vi "TargetArduinoControlled.vi"() -> ()   [LabVIEW 2013]
uses:
  <vilib>/Instr/_visa.llb/VISA Configure Serial Port (Instr).vi
  <vilib>/express/express arith-compare/Formula/XNode/ExpressFormulaBlockNode.xnode
panel:
  out "Tension de commande (V)":dbl
  out "Phidget device handle 2":i64
  out "Phidget device handle":i64
  out "Phidget Error Cluster":errorcluster
  in  "ArduinoSpeedSelect":i8(slide) scale=0.0..3.0
  out "Arduino Answer":string
  in  "Test Function":bool
  in  "Calibrate":bool
  out "shot until":dbl
  out "Target":cluster{dbl, dbl}(knob)={0.0, 360.0} scale=0.0..360.0
  in  "Shoot":bool
  out "TargetPosition":dbl
  out "moving":bool
  in  "Continious Slow motion":bool
  in  "Reset Shots":bool
  in  "Stop":bool
  in  "VISA resource name":refnum<visa-resource-name>="COM7" caption="Arduino Communication Port"
  out "shooting length (mm)":dbl
  in  "Sequence (ms)":i16
  in  "start rotation":bool
  in  "rotation stop":bool
  out "shooting radius (microns)":dbl
  in  "target radius":dbl=50600.0
  in  "Spot_spacing_µm":dbl=100.0
  in  "Position edge (microns)":dbl=-8706.0
  in  "Position Target (microns)":dbl=14475.0
  out "SpeedTarget  (rounds/s)":dbl
  out "tension envoyée V":dbl
  in  "event trigger":bool
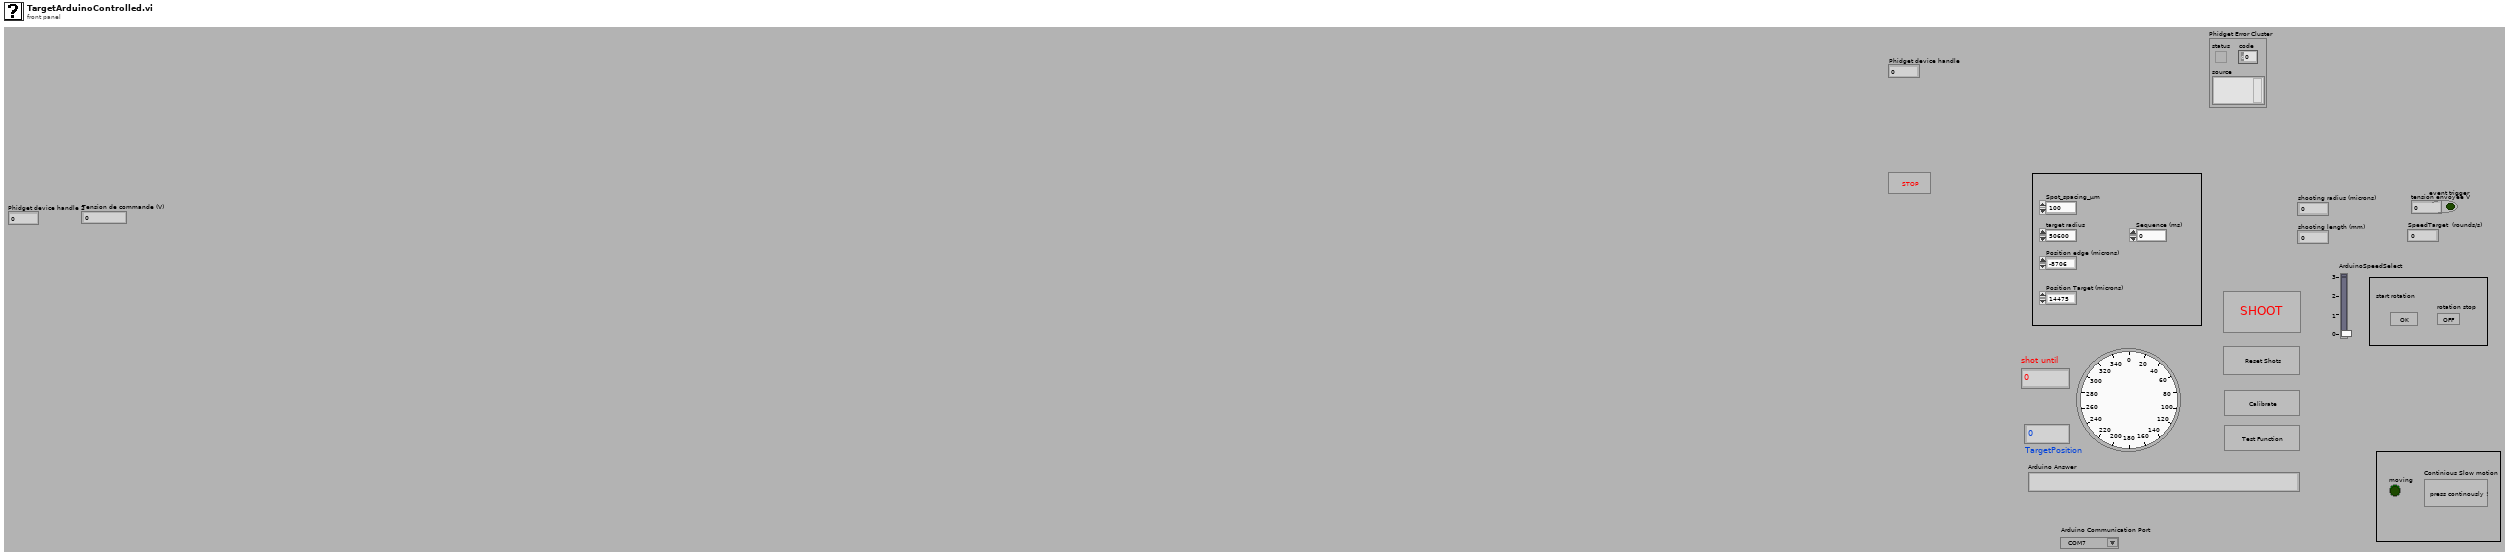
[diagram p1: front panel]
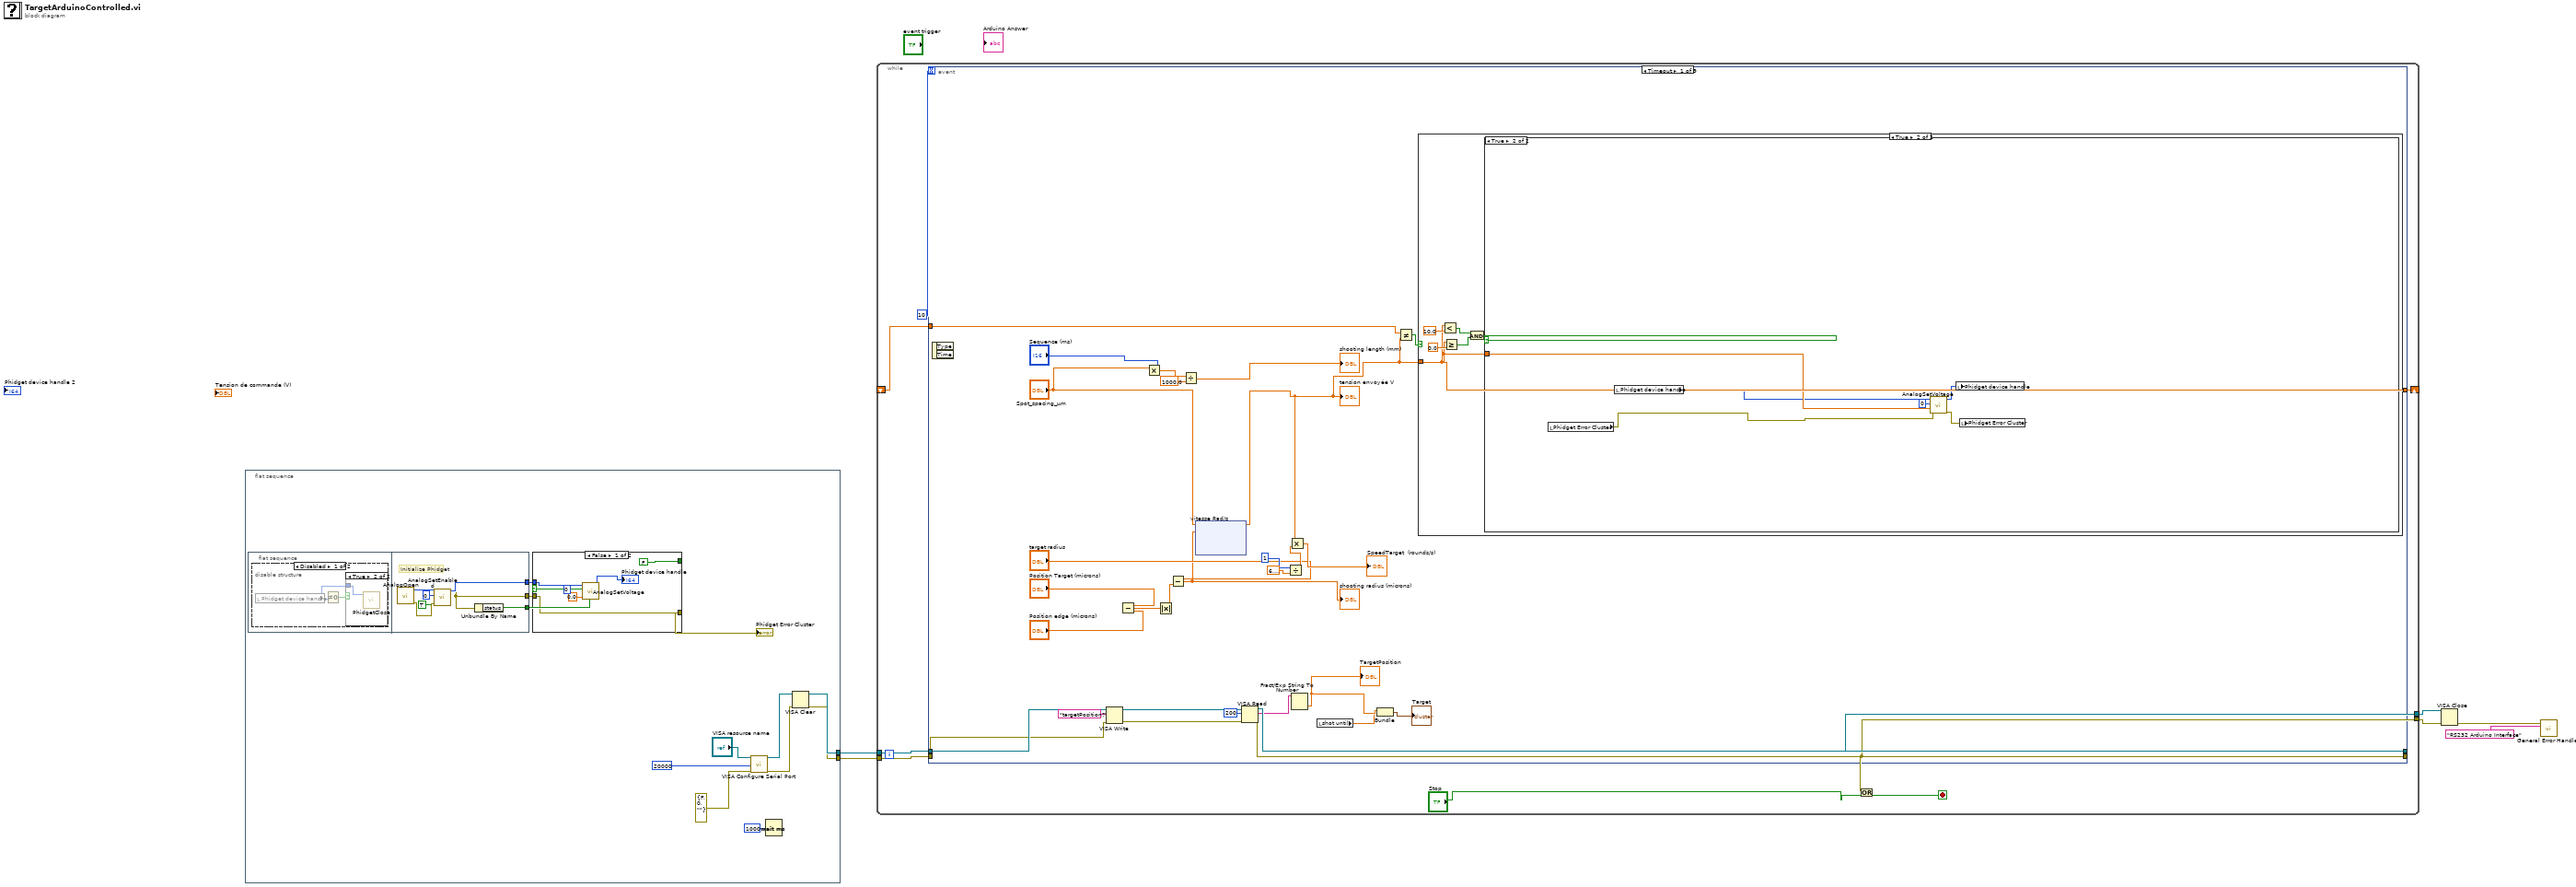
[diagram p0: block diagram]
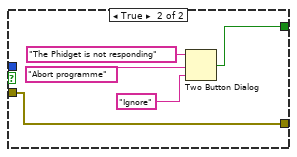
[diagram p2: hidden frame]
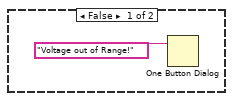
[diagram p6: hidden frame]
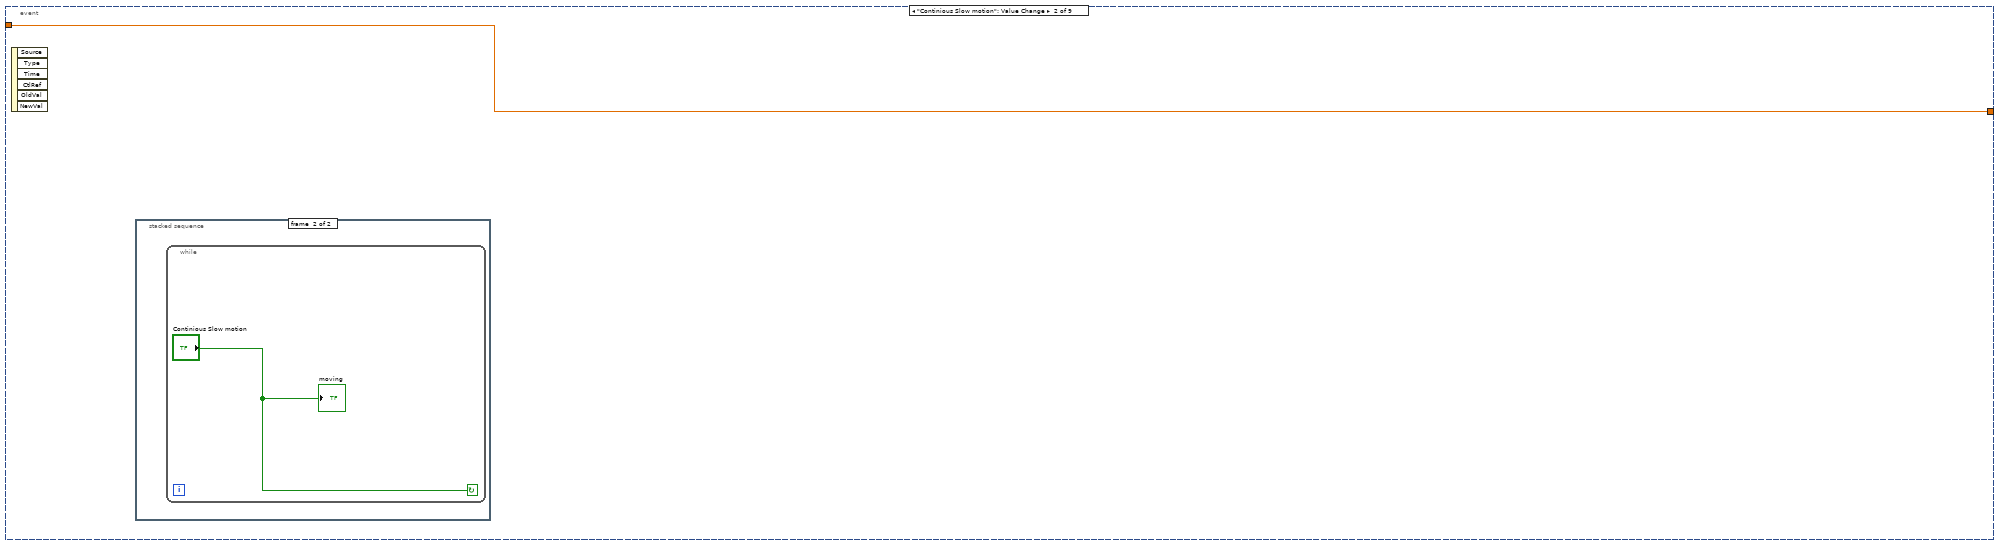
[diagram p7: hidden frame]
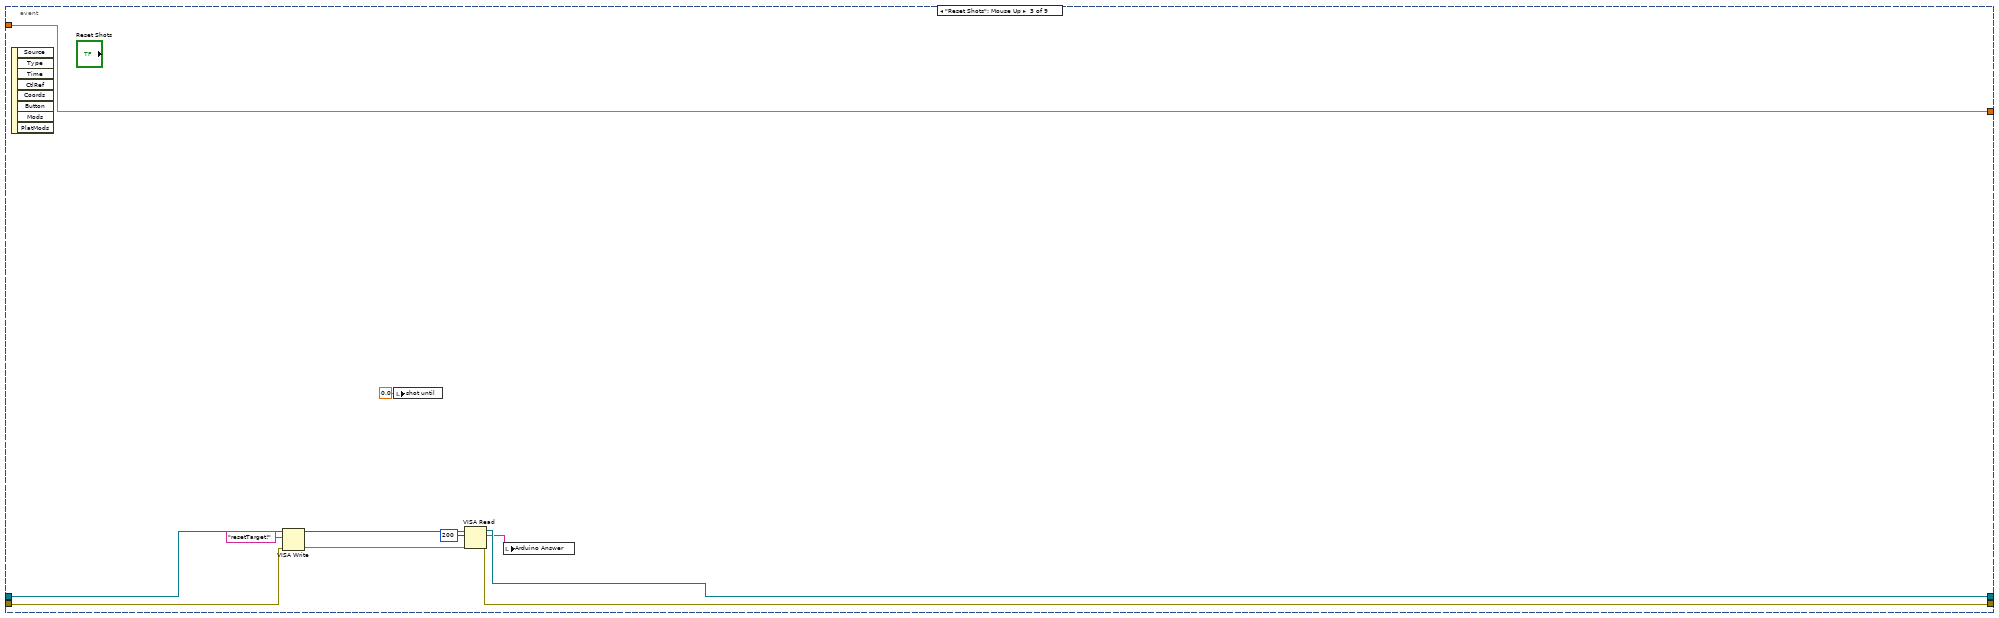
[diagram p9: hidden frame]
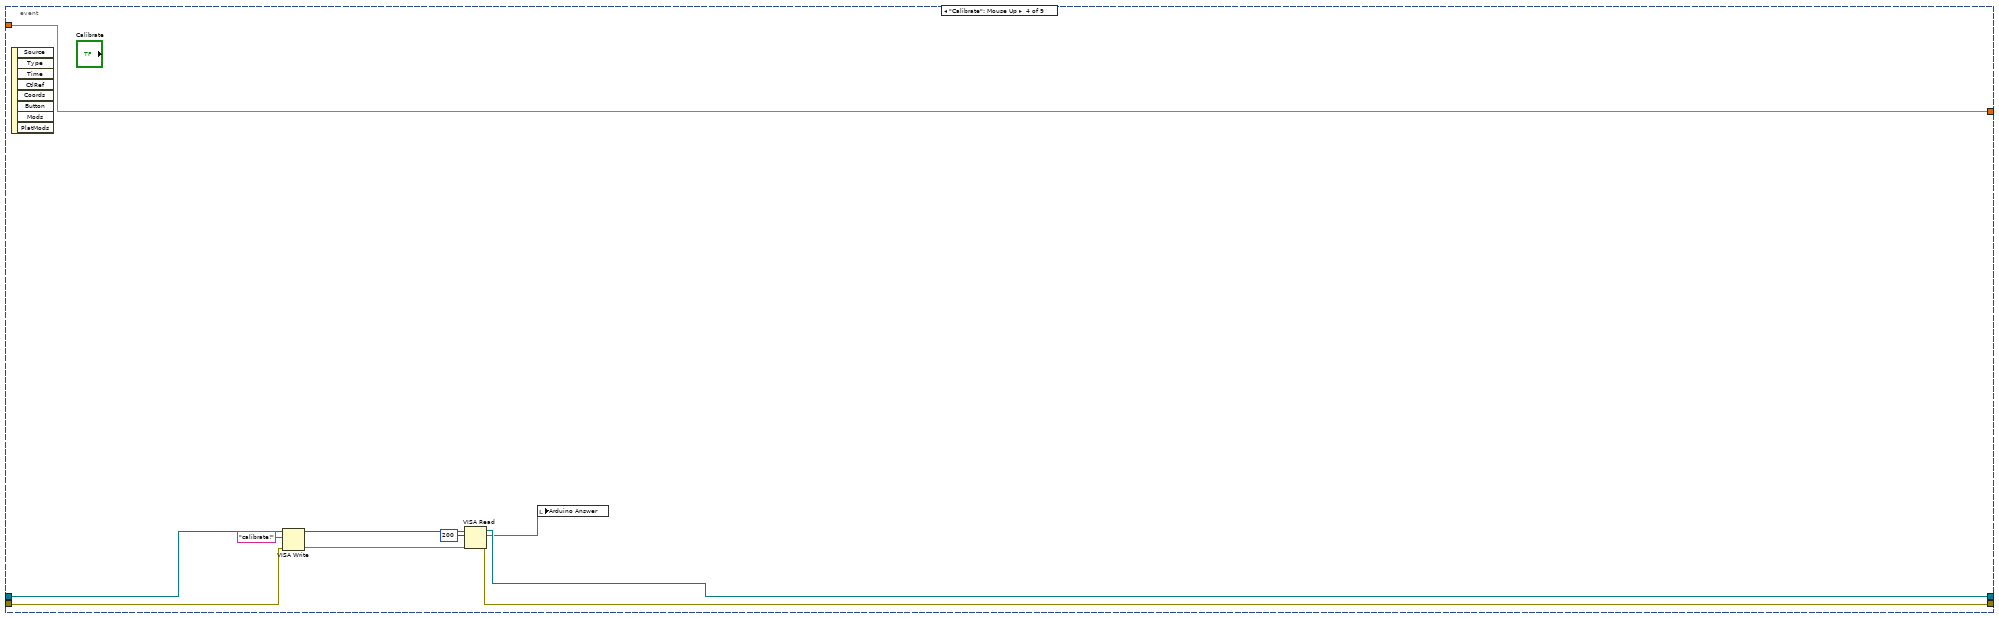
[diagram p10: hidden frame]
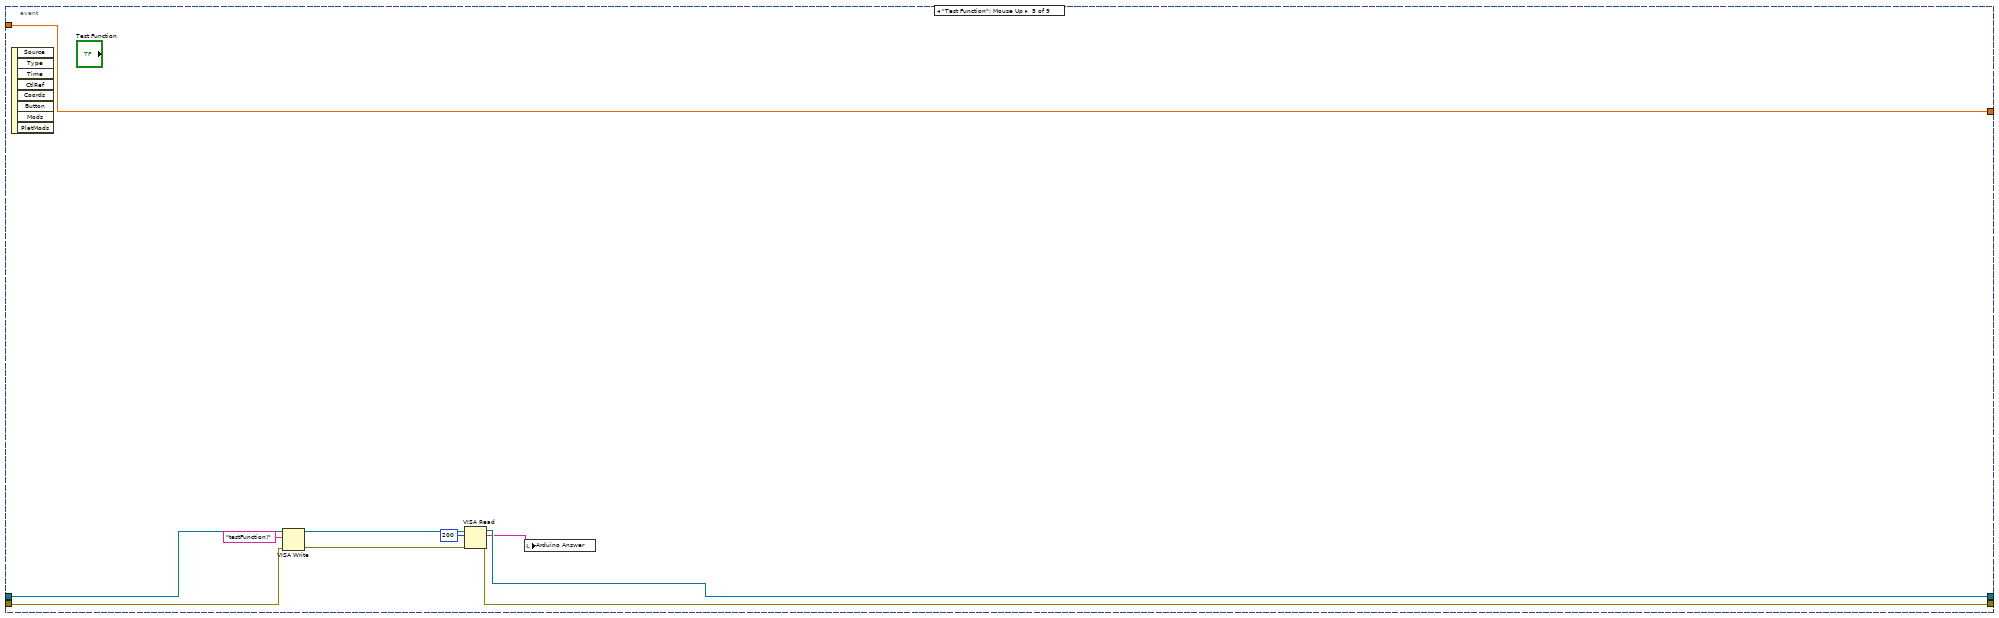
[diagram p11: hidden frame]
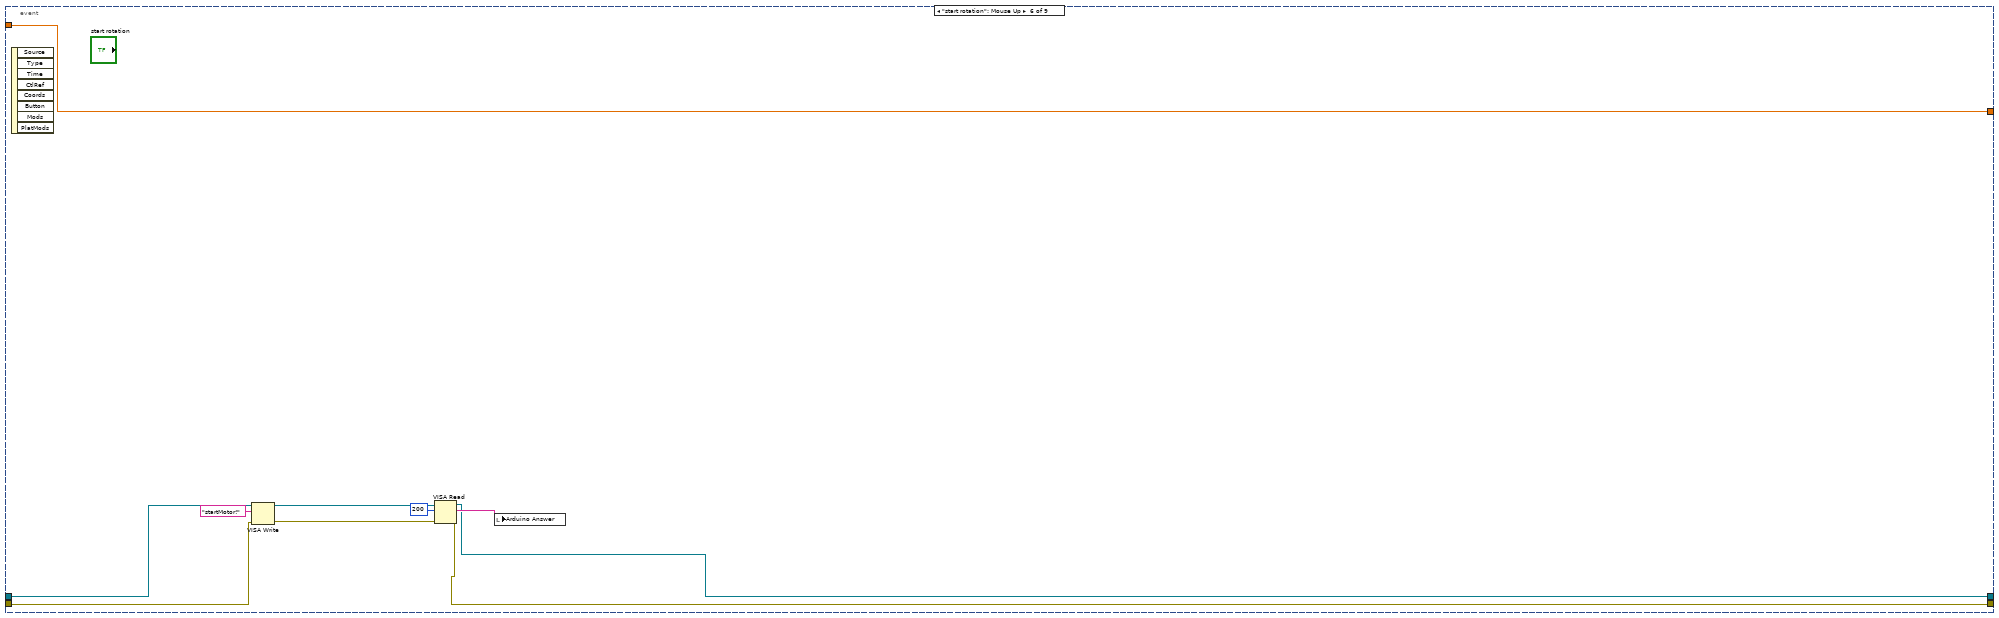
[diagram p12: hidden frame]
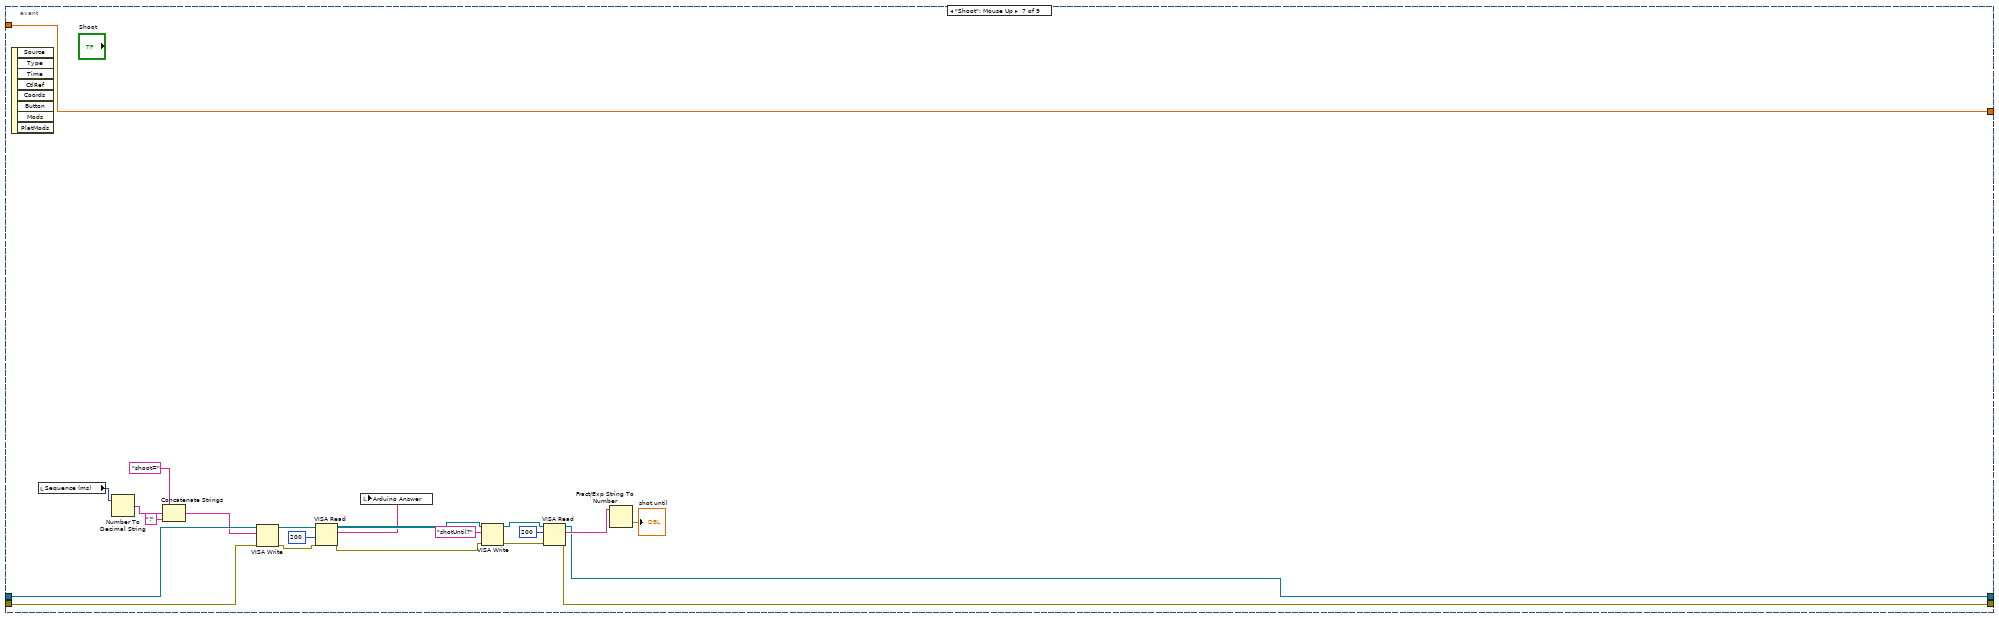
[diagram p13: hidden frame]
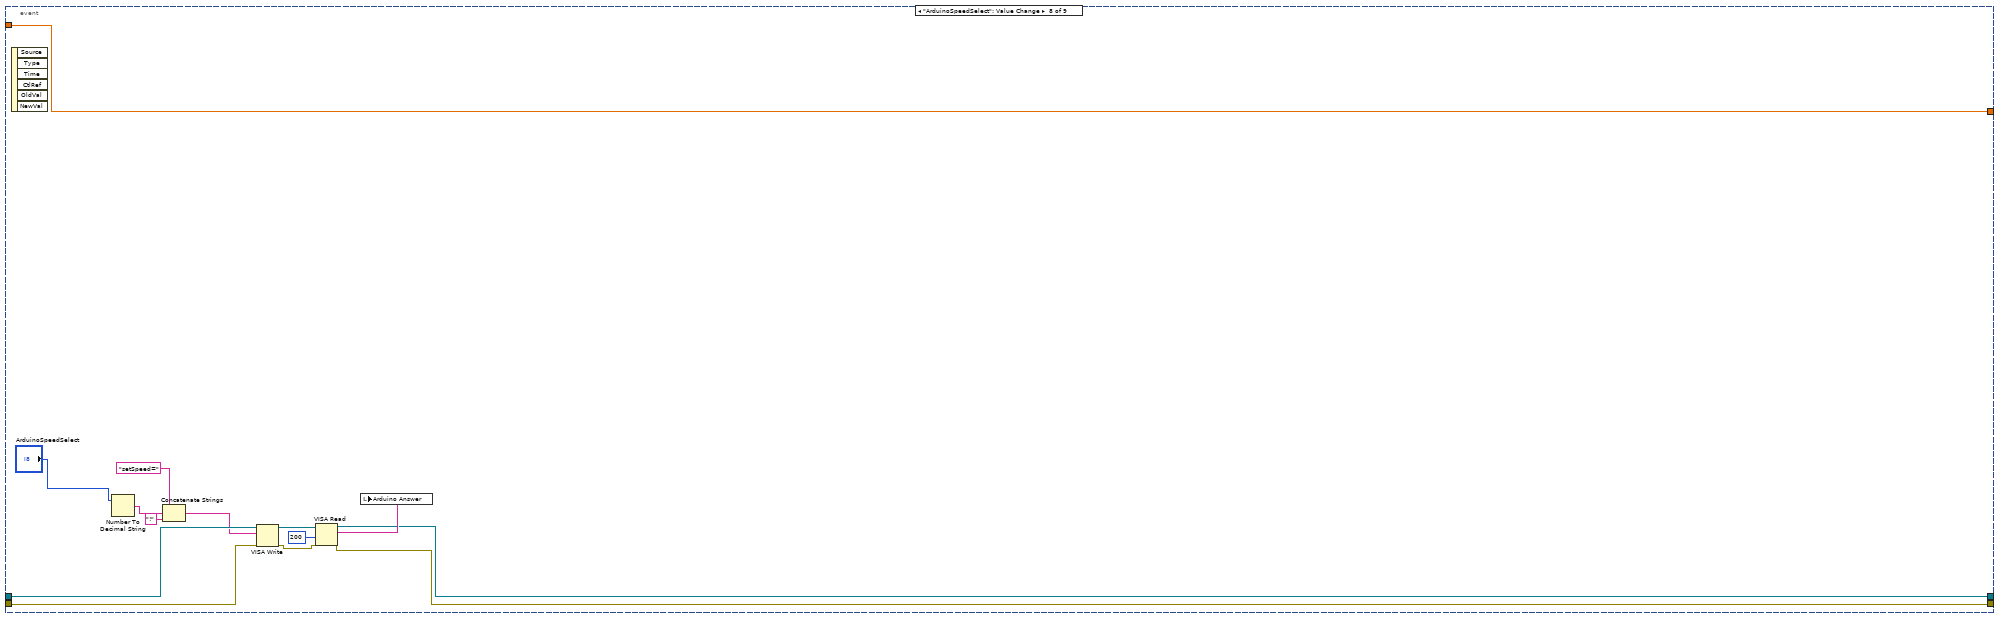
[diagram p14: hidden frame]
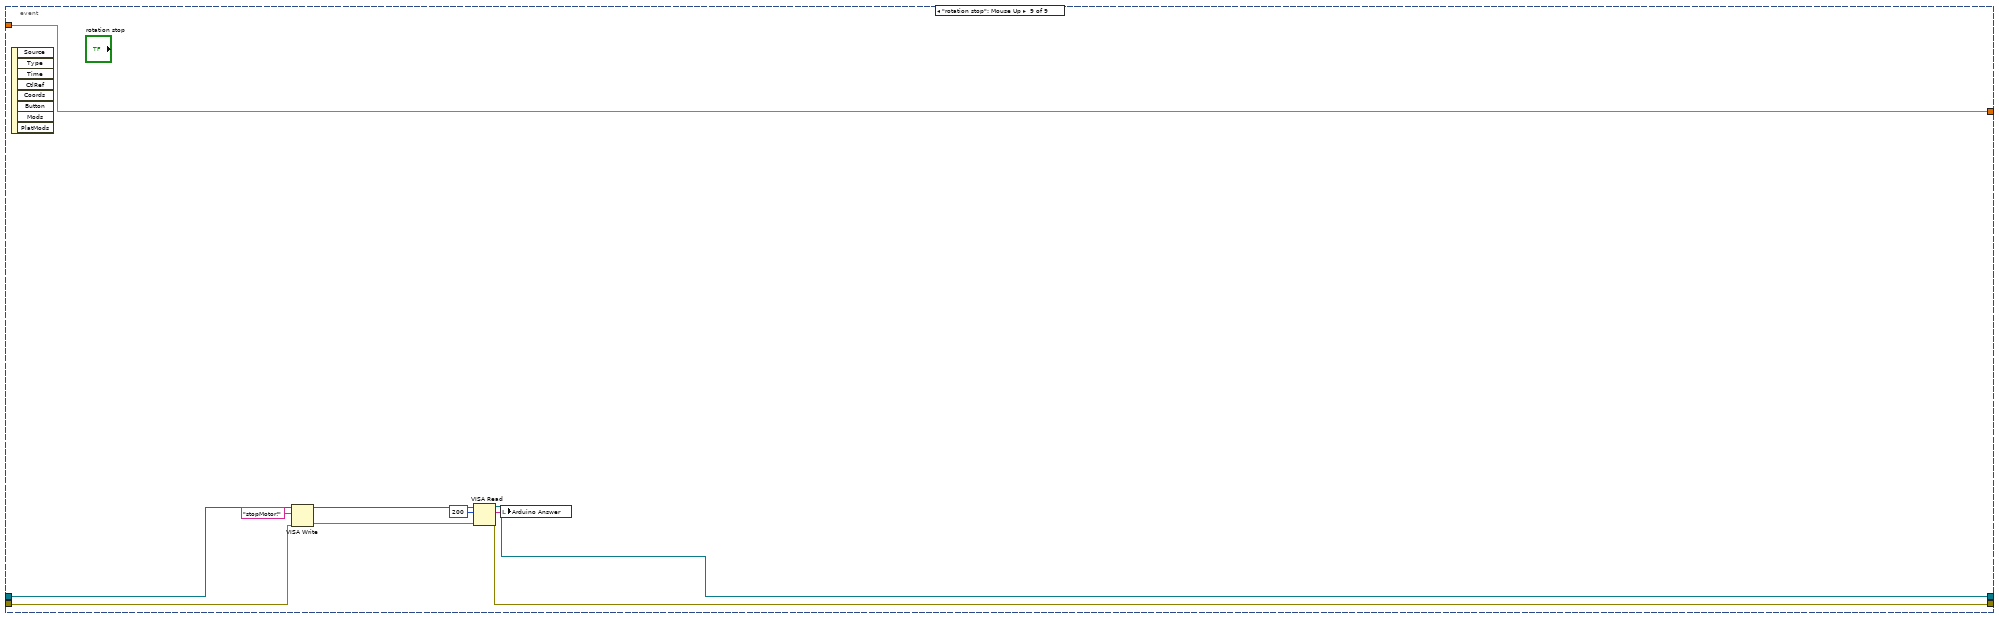
[diagram p15: hidden frame]
diagram:
  n1 = flat-sequence {
    tunnel: [w13] -> w6
    tunnel: [w12] -> w5
    frame #0 {
      n2 = flat-sequence {
        tunnel: [w35] -> w8
        tunnel: [w34] -> w9
        tunnel: [w33] -> w10
        frame #0 {
          n3 = disable-structure shown="Disabled" {
            frame Disabled {
              n4 = local read "Phidget device handle"() -> (w30:i64)
              n5 = Not Equal To 0?(x=w30) -> (x != 0?=w31:bool)
              n6 = case shown="True" w31 {
                tunnel: w30 -> [_ w32]
                frame False {
                }
                frame True {
                  n7 = call "PhidgetClose.vi"("Device In"=w32) -> ()  [unwired: 10 in, 1 out]
                }
              }
            }
            frame Enabled {
            }
          }
        }
        frame #1 {
          # "Initialize Phidget"
          n8 = call "AnalogOpen.vi"() -> ("error out"=w39:errorcluster, "Device Out"=w36:i32)  [unwired: 8 in, 2 out]
          n9 = call "AnalogSetEnabled.vi"("error in (no error)"=w39, "SetEnabled"=TRUE, "index"=0, "Device In"=w36) -> ("error out"=w33:errorcluster, "Device Out"=w34:i32)  [unwired: 5 in]
          n10 = Unbundle By Name(w33) -> ("status"=w35:bool)
        }
      }
      n11 = case shown="False" w8 {
        tunnel: [FALSE w26] -> _
        tunnel: w9 -> [w23 _]
        tunnel: w10 -> [w21 w25]
        tunnel: [w21 w25] -> w7
        frame False {
          n12 = call "AnalogSetVoltage.vi"("voltage"=0.0, "index"=0, "Device In"=w23) -> ("Device Out"=→"Phidget device handle":i32)  [unwired: 6 in, 1 out]
        }
        frame True {
          n13 = Two Button Dialog(message="The Phidget is not responding", 1:"Ignore" ("Nom du bouton V (\"OK\")"), 2:"Abort programme" ("Nom du bouton V (\"OK\")")) -> (T button?=w26:bool)
        }
      }
      "Phidget Error Cluster" <- w7
      n14 = call-poly "VISA Configure Serial Port"("VISA resource name"="VISA resource name", "timeout (10sec)"=u32 20000, "error in (no error)"=errorcluster {"status"=FALSE, "code"=0, "source"=""}) -> ("VISA resource name out"=w16:refnum<visa-resource-name>, "error out"=w14:errorcluster)  [unwired: 11 in]
      n15 = Wait (ms)(milliseconds to wait=u32 1000 ("attente (ms)")) -> ()  [unwired: 1 out]
      n16 = VISA Clear(VISA resource name=w16, error in (no error)=w14) -> (VISA resource name out=w13:refnum<visa-resource-name>, error out=w12:errorcluster)
    }
  }
  n17 = while {
    tunnel: w6 -> [w46]
    tunnel: w5 -> [w45]
    tunnel: [w42] -> w3
    tunnel: [w44] -> w2
    shift-right: [w41] -> _
    shift-left: _ -> [w40]
    stop <- w43 stop-if-true
    n18 = event shown="[0] Timeout" {
      selector: _ -> [_ _ _ _ _ _ _ _ _]
      dyn-events: _ -> [_ _ _ _ _ _ _ _ _]
      timeout: 10 -> [_ _ _ _ _ _ _ _ _]
      tunnel: w46 -> [w64 _ w110 w120 w130 w139 w162 w180 w183]
      tunnel: [w62 _ w108 w118 w128 w137 w164 w170 w185] -> w44
      tunnel: [w61 _ w107 w117 w127 w136 w163 w169 w184] -> w42
      tunnel: w45 -> [w59 _ w109 w119 w129 w138 w161 w179 w182]
      tunnel: [w50 w102 w104 w115 w125 w135 w145 w167 w181] -> w41
      tunnel: w40 -> [w51 w102 w104 w115 w125 w135 w145 w167 w181]
      event Timeout {
        n19 = event-data() -> ()  [unwired: 1 in, 2 out]
        n20 = VISA Write(VISA resource name=w64, write buffer="targetPosition?" ("buffer à écrire"), error in (no error)=w59) -> (VISA resource name out=w63:refnum<visa-resource-name>, error out=w60:errorcluster)  [unwired: 1 out]
        n21 = Subtract(x="Position Target (microns)", y="Position edge (microns)") -> (x-y=w73:dbl)
        n22 = Multiply(x="Spot_spacing_µm", y="Sequence (ms)") -> (x*y=w68:dbl)
        n23 = Absolute Value(x=w73) -> (abs(x)=w72:dbl)
        n24 = Subtract(x="target radius", y=w72) -> (x-y=w65:dbl)
        "shooting radius (microns)" <- w65
        n25 = Divide(x=w68, y=1000.0) -> (x/y=→"shooting length (mm)":dbl)
        n26 = xnode ("vitesse Rad/s")("Spot_spacing_µm"="Spot_spacing_µm", "Radius_µm"=w65) -> ("Result"=w50:dbl)  [unwired: 1 in, 1 out]
        "tension envoyée V" <- w50
        n27 = VISA Read(VISA resource name=w63, byte count=u32 200 ("nombre d'octets"), error in (no error)=w60) -> (VISA resource name out=w62:refnum<visa-resource-name>, read buffer=w56:string, error out=w61:errorcluster)  [unwired: 1 out]
        n28 = Divide(x=1, y=6.283185307179586) -> (x/y=w76:dbl)
        n29 = Multiply(x=w50, y=w76) -> (x*y=→"SpeedTarget  (rounds/s)":dbl)
        n30 = Fract/Exp String To Number(string=w56) -> (number=w55:dbl)  [unwired: 3 in, 1 out]
        "TargetPosition" <- w55
        n31 = local read "shot until"() -> (w54:dbl)
        n32 = Bundle(w55, "shot until"=w54) -> (→"Target":cluster{dbl, "shot until":dbl})  [unwired: 1 in]
        n33 = Not Equal?(x=w51, y=w50) -> (x != y?=w49:bool)
        n34 = case shown="True" w49 {
          tunnel: w50 -> [_ w79]
          frame False {
          }
          frame True {
            n35 = Less?(x=w79, y=10.0) -> (x < y?=w82:bool)
            n36 = Greater Or Equal?(x=w79, y=0.0) -> (x >= y?=w81:bool)
            n37 = And(x=w82, y=w81) -> (x .and. y?=w80:bool)
            n38 = case shown="True" w80 {
              tunnel: w79 -> [_ w91]
              frame False {
                n39 = One Button Dialog(message="Voltage out of Range!") -> ()  [unwired: 1 in, 1 out]
              }
              frame True {
                n40 = local read "Phidget Error Cluster"() -> (w86:errorcluster)
                n41 = local read "Phidget device handle"() -> (w87:i64)
                n42 = call "AnalogSetVoltage.vi"("error in (no error)"=w86, "voltage"=w91, "index"=0, "Device In"=w87) -> ("error out"=w88:errorcluster, "Device Out"=w89:i32)  [unwired: 5 in]
                n43 = local write "Phidget device handle"(w89) -> ()
                n44 = local write "Phidget Error Cluster"(w88) -> ()
              }
            }
          }
        }
      }
      event "Continious Slow motion": Value Change {
        n45 = event-data() -> ()  [unwired: 1 in, 6 out]
        n46 = stacked-sequence {
          frame #0 {
          }
          frame #1 {
            n47 = while {
              stop <- "Continious Slow motion" continue-if-true
              "moving" <- "Continious Slow motion"
            }
          }
        }
      }
      event "Reset Shots": Mouse Up {
        n48 = event-data() -> ()  [unwired: 1 in, 8 out]
        n49 = VISA Write(VISA resource name=w110, write buffer="resetTarget!" ("buffer à écrire"), error in (no error)=w109) -> (VISA resource name out=w114:refnum<visa-resource-name>, error out=w113:errorcluster)  [unwired: 1 out]
        n50 = local write "shot until"(0.0 ("shot until")) -> ()
        n51 = VISA Read(VISA resource name=w114, byte count=u32 200 ("nombre d'octets"), error in (no error)=w113) -> (VISA resource name out=w108:refnum<visa-resource-name>, read buffer=w105:string, error out=w107:errorcluster)  [unwired: 1 out]
        n52 = local write "Arduino Answer"(w105) -> ()
      }
      event "Calibrate": Mouse Up {
        n53 = event-data() -> ()  [unwired: 1 in, 8 out]
        n54 = VISA Write(VISA resource name=w120, write buffer="calibrate!" ("buffer à écrire"), error in (no error)=w119) -> (VISA resource name out=w124:refnum<visa-resource-name>, error out=w123:errorcluster)  [unwired: 1 out]
        n55 = VISA Read(VISA resource name=w124, byte count=u32 200 ("nombre d'octets"), error in (no error)=w123) -> (VISA resource name out=w118:refnum<visa-resource-name>, read buffer=w116:string, error out=w117:errorcluster)  [unwired: 1 out]
        n56 = local write "Arduino Answer"(w116) -> ()
      }
      event "Test Function": Mouse Up {
        n57 = event-data() -> ()  [unwired: 1 in, 8 out]
        n58 = VISA Write(VISA resource name=w130, write buffer="testFunction!" ("buffer à écrire"), error in (no error)=w129) -> (VISA resource name out=w134:refnum<visa-resource-name>, error out=w133:errorcluster)  [unwired: 1 out]
        n59 = VISA Read(VISA resource name=w134, byte count=u32 200 ("nombre d'octets"), error in (no error)=w133) -> (VISA resource name out=w128:refnum<visa-resource-name>, read buffer=w126:string, error out=w127:errorcluster)  [unwired: 1 out]
        n60 = local write "Arduino Answer"(w126) -> ()
      }
      event "start rotation": Mouse Up {
        n61 = event-data() -> ()  [unwired: 1 in, 8 out]
        n62 = VISA Write(VISA resource name=w139, write buffer="startMotor!" ("buffer à écrire"), error in (no error)=w138) -> (VISA resource name out=w144:refnum<visa-resource-name>, error out=w143:errorcluster)  [unwired: 1 out]
        n63 = VISA Read(VISA resource name=w144, byte count=u32 200 ("nombre d'octets"), error in (no error)=w143) -> (VISA resource name out=w137:refnum<visa-resource-name>, read buffer=w140:string, error out=w136:errorcluster)  [unwired: 1 out]
        n64 = local write "Arduino Answer"(w140) -> ()
      }
      event "Shoot": Mouse Up {
        n65 = event-data() -> ()  [unwired: 1 in, 8 out]
        n66 = local read "Sequence (ms)"() -> (w156:i16)
        n67 = Number To Decimal String(number=w156) -> (decimal integer string=w155:string)  [unwired: 1 in]
        n68 = Concatenate Strings("shoot=" ("buffer à écrire"), w155, "!" ("chaîne")) -> (w153:string)
        n69 = VISA Write(VISA resource name=w162, write buffer=w153, error in (no error)=w161) -> (VISA resource name out=w159:refnum<visa-resource-name>, error out=w158:errorcluster)  [unwired: 1 out]
        n70 = VISA Read(VISA resource name=w159, byte count=u32 200 ("nombre d'octets"), error in (no error)=w158) -> (VISA resource name out=w148:refnum<visa-resource-name>, read buffer=w146:string, error out=w149:errorcluster)  [unwired: 1 out]
        n71 = local write "Arduino Answer"(w146) -> ()
        n72 = VISA Write(VISA resource name=w148, write buffer="shotUntil?" ("buffer à écrire"), error in (no error)=w149) -> (VISA resource name out=w151:refnum<visa-resource-name>, error out=w150:errorcluster)  [unwired: 1 out]
        n73 = VISA Read(VISA resource name=w151, byte count=u32 200 ("nombre d'octets"), error in (no error)=w150) -> (VISA resource name out=w164:refnum<visa-resource-name>, read buffer=w165:string, error out=w163:errorcluster)  [unwired: 1 out]
        n74 = Fract/Exp String To Number(string=w165) -> (number=→"shot until":dbl)  [unwired: 3 in, 1 out]
      }
      event "ArduinoSpeedSelect": Value Change {
        n75 = event-data() -> ()  [unwired: 1 in, 6 out]
        n76 = Number To Decimal String(number="ArduinoSpeedSelect") -> (decimal integer string=w176:string)  [unwired: 1 in]
        n77 = Concatenate Strings("setSpeed=" ("buffer à écrire"), w176, "!" ("chaîne")) -> (w174:string)
        n78 = VISA Write(VISA resource name=w180, write buffer=w174, error in (no error)=w179) -> (VISA resource name out=w168:refnum<visa-resource-name>, error out=w177:errorcluster)  [unwired: 1 out]
        n79 = VISA Read(VISA resource name=w168, byte count=u32 200 ("nombre d'octets"), error in (no error)=w177) -> (VISA resource name out=w170:refnum<visa-resource-name>, read buffer=w172:string, error out=w169:errorcluster)  [unwired: 1 out]
        n80 = local write "Arduino Answer"(w172) -> ()
      }
      event "rotation stop": Mouse Up {
        n81 = event-data() -> ()  [unwired: 1 in, 8 out]
        n82 = VISA Write(VISA resource name=w183, write buffer="stopMotor!" ("buffer à écrire"), error in (no error)=w182) -> (VISA resource name out=w190:refnum<visa-resource-name>, error out=w189:errorcluster)  [unwired: 1 out]
        n83 = VISA Read(VISA resource name=w190, byte count=u32 200 ("nombre d'octets"), error in (no error)=w189) -> (VISA resource name out=w185:refnum<visa-resource-name>, read buffer=w186:string, error out=w184:errorcluster)  [unwired: 1 out]
        n84 = local write "Arduino Answer"(w186) -> ()
      }
    }
    n85 = Or(x=w42, y="Stop") -> (x .or. y?=w43:bool)
  }
  n86 = VISA Close(VISA resource name=w2, error in (no error)=w3) -> (error out=w4:errorcluster)
  n87 = call <vilib>:"General Error Handler.vi"("[error source] (\" \")"="RS232 Arduino Interface" ("[error source] (\" \")"), "error in (no error)"=w4) -> ()  [unwired: 9 in, 5 out]
